vi "DTW.vi"(8 "Reference Sequence":T1, 11 "Test Sequence":T1) -> (1 "Cost":dbl)   [LabVIEW 2012]
uses:
  <vilib>/silver_ctls/ArrayMatrixCluster/Real Matrix NI_Silver.ctl
  <vilib>/imath/engines/lvmath2/RunTimeEngine/ErrorHandling/NIMS_Finalize Error.vi
  <vilib>/imath/engines/lvmath2/RunTimeEngine/ReplaceToken/NIMS_Replace - Check Row.vi
  <instcachedir>/0/NIMS_Replace - Check Row_8C35B66FE73A429EAC382AAA935851F0.lvgen/NIMS_Replace - Check Row_8C35B66FE73A429EAC382AAA935851F0_000.vi
  <vilib>/imath/engines/lvmath2/RunTimeEngine/ReplaceToken/NIMS_Replace - Check Column.vi
  <instcachedir>/0/NIMS_Replace - Check Column_F9ADE87E459D46779ACFAE3AFB317B9B.lvgen/NIMS_Replace - Check Column_F9ADE87E459D46779ACFAE3AFB317B9B_001.vi
  <vilib>/imath/engines/lvmath2/RunTimeEngine/VariableToken/Read/NIMS_Get Elements - SorM(_,_) - Check - Check.vi
  <instcachedir>/0/NIMS_Get Elements - SorM(_,_) - Check - Check_3492346BAECA4EC09E2016EA7EC0034B.lvgen/NIMS_Get Elements - SorM(_,_) - Check - Check_3492346BAECA4EC09E2016EA7EC0034B_001.vi
  <vilib>/imath/engines/lvmath2/RunTimeEngine/ReplaceToken/NIMS_Replace - Size Check M(_,_)=S.vi
  <instcachedir>/0/NIMS_Replace - Size Check M(_,_)=S_0CFA00F12BB840EDA61E43D782562782.lvgen/NIMS_Replace - Size Check M(_,_)=S_0CFA00F12BB840EDA61E43D782562782_000.vi
  <vilib>/imath/engines/lvmath2/RunTimeEngine/ReplaceToken/NIMS_Replace - M(S,S)=S.vi
  <instcachedir>/0/NIMS_Replace - M(S,S)=S_59120E3D3E804D63A1B2B7FDD4B95F55.lvgen/NIMS_Replace - M(S,S)=S_59120E3D3E804D63A1B2B7FDD4B95F55_000.vi
  <vilib>/imath/engines/lvmath2/RunTimeEngine/ErrorHandling/NIMS_Create Error From Enums.vi
  <vilib>/imath/engines/lvmath2/RunTimeEngine/RangeToken/NIMS_Range_R2 - Integer.vi
  <instcachedir>/0/NIMS_Range_R2 - Integer_CD92A44154CA48D58B2F3E711AB114DB.lvgen/NIMS_Range_R2 - Integer_CD92A44154CA48D58B2F3E711AB114DB_000.vi
  <vilib>/imath/engines/lvmath2/RunTimeEngine/NodeEndStatement/NIMS_NodeEndStatement_Output.vi
  <instcachedir>/0/NIMS_NodeEndStatement_Output_53EC0D466D134D7ABD903AC30B43404B.lvgen/NIMS_NodeEndStatement_Output_53EC0D466D134D7ABD903AC30B43404B_001.vi
  <vilib>/imath/engines/lvmath2/RunTimeEngine/CommandStatement/MC_CommandStatement_break.vi
  <vilib>/imath/engines/lvmath2/RunTimeEngine/BuiltInFunctions/min/1 input/NIMS_min(RV).vi
  <instcachedir>/0/NIMS_min(RV)_EE2DD3E2888846108C5160A664B67832.lvgen/NIMS_min(RV)_EE2DD3E2888846108C5160A664B67832_000.vi
  <vilib>/imathl/engines/lvmath/Functions/Error Handling/Create Error.vi
panel:
  out "Local Cost Matrix":dbl[][](array[numeric])
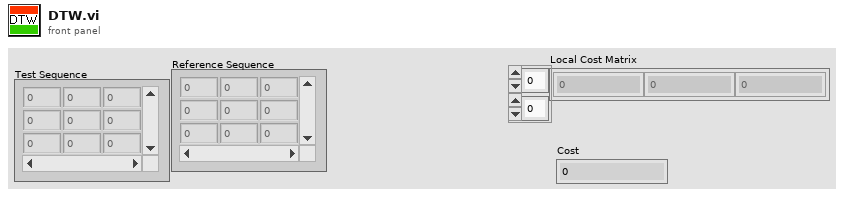
[diagram p1: front panel]
types:
  T1 = typedef "Real Matrix NI_Silver.ctl" = dbl[][]
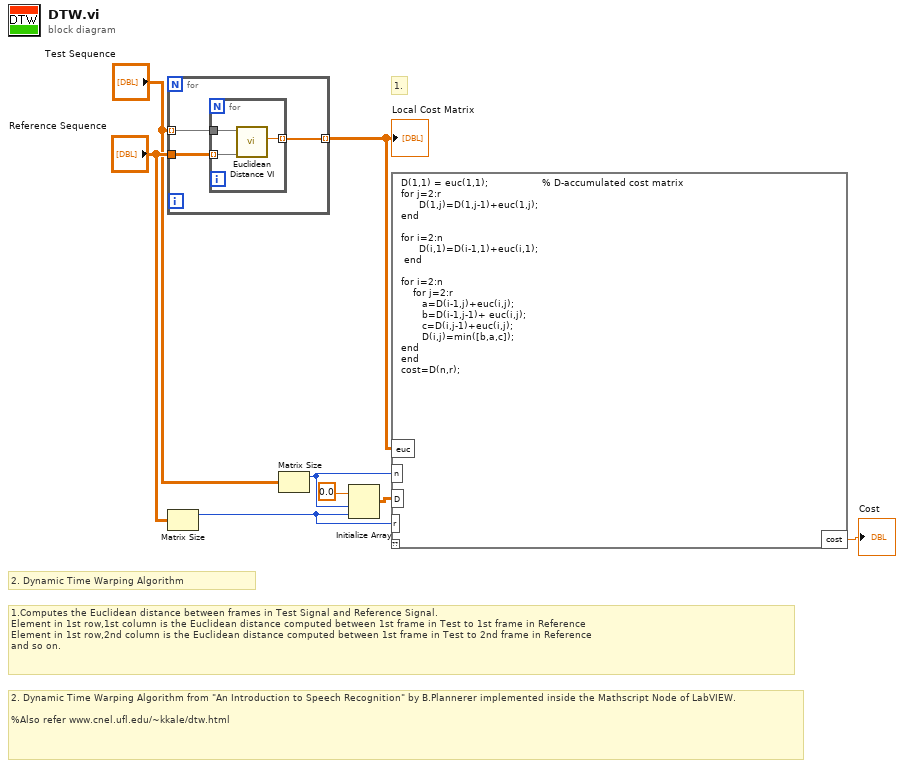
[diagram p0: block diagram]
diagram:
  # "2. Dynamic Time Warping Algorithm from \"An Introduction to Speech Recognition\" by B.Plannerer implemented inside the Mathscript Node of LabVIEW.\n\n%Also refer www.cnel.ufl.edu/~kkale/dtw.html"
  # "1.Computes the Euclidean distance between frames in Test Signal and Reference Signal.\nElement in 1st row,1st column is the Euclidean distance computed between 1st frame in Test to 1st frame in Reference\nElement in 1st row,2nd column is the Euclidean distance computed between 1st frame in Test to 2nd frame in Reference\nand so on."
  # "1."
  # "2. Dynamic Time Warping Algorithm"
  n1 = for {
    tunnel: "Test Sequence" -> [w10] mode=indexing
    tunnel: "Reference Sequence" -> [w11]
    tunnel: [w9] -> w4 mode=indexing
    n2 = for {
      tunnel: w11 -> [w13] mode=indexing
      tunnel: w10 -> [w14]
      tunnel: [w12] -> w9 mode=indexing
      n3 = call "Euclidean Distance VI.vi"("Reference"=w13, "Test"=w14) -> ("Dist"=w12:dbl)  [unwired: 9 in]
    }
  }
  "Local Cost Matrix" <- w4
  n4 = Matrix Size(0:"Reference Sequence") -> (1:w3:i32)  [unwired: 1 out]
  n5 = Matrix Size(0:"Test Sequence") -> (1:w5:i32)  [unwired: 1 out]
  n6 = Initialize Array(0.0 ("element"), w5, w3) -> (w1:dbl[][])
  n7 = mathscript code="D(1,1) = euc(1,1);                  % D-accumulated cost matrix\nfor j=2:r\n      D(1,j)=D(1,j-1)+euc(1,j);\nend\n\nfor i=2:n\n      D(i,1)=D(i-1,1)+euc(i,1);\n end\n\nfor i=2:n\n    for j=2:r     \n       a=D(i-1,j)+euc(i,j);\n       b=D(i-1,j-1)+ euc(i,j);\n       c=D(i,j-1)+euc(i,j);\n       D(i,j)=min([b,a,c]);\nend\nend\ncost=D(n,r);"("euc"=w4, "n"=w5, "r"=w3, "D"=w1) -> ("cost"=→"Cost":dbl)  [unwired: 1 in, 1 out]
